vi "movemotor.vi"(8 "error in (no error)":errorcluster, 10 "motor voltage":dbl, 11 "hardware v1 in":refnum<class "hardware v1.lvclass">) -> (0 "error out":errorcluster, 3 "hardware v1 out":refnum<class "hardware v1.lvclass">)   [LabVIEW 2015, in "hardware v1.lvclass"]
uses:
  hardware v1.lvclass
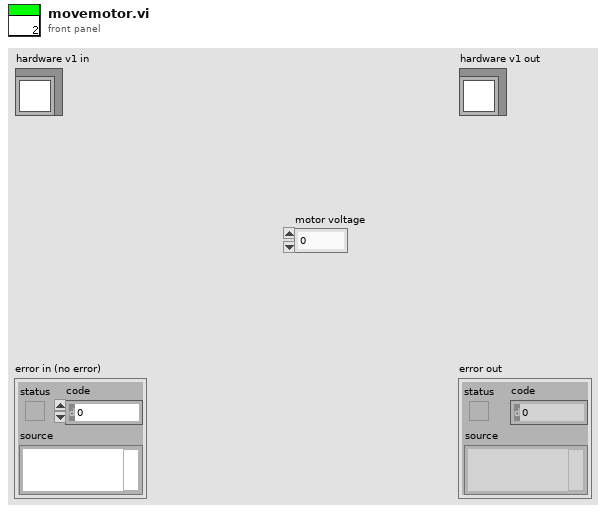
[diagram p1: front panel]
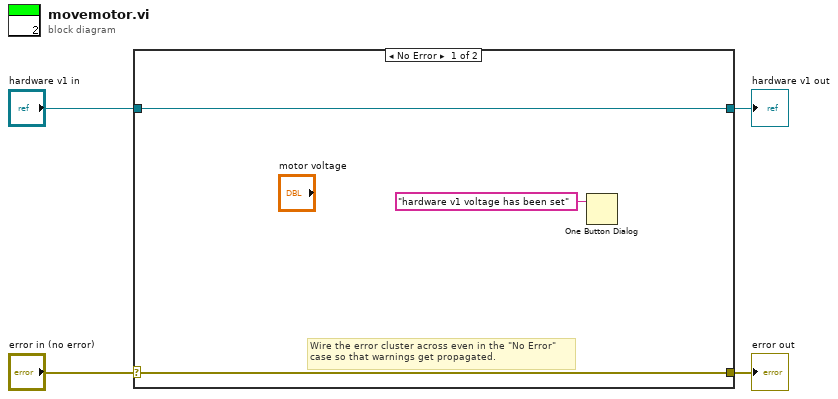
[diagram p0: block diagram]
diagram:
  n1 = case shown="No Error" "error in (no error)" {
    selector: "error in (no error)" -> [w6 w9]
    tunnel: [w6 w9] -> w3
    tunnel: [w7 w8] -> w1
    tunnel: "hardware v1 in" -> [w7 w8]
    frame No Error {
      # "Wire the error cluster across even in the \"No Error\"\ncase so that warnings get propagated."
      n2 = One Button Dialog(message="hardware v1 voltage has been set") -> ()  [unwired: 1 in, 1 out]
    }
    frame Error {
    }
  }
  "error out" <- w3
  "hardware v1 out" <- w1
